vi "Set Helper Text.vi"(8 "error in (no error)":errorcluster, 10 "Helper Text":string, 11 "Filled Text Fields in":refnum<class "Filled Text Fields.lvclass">) -> (0 "error out":errorcluster, 3 "Filled Text Fields out":refnum<class "Filled Text Fields.lvclass">)   [LabVIEW 2017, in "Filled Text Fields.lvlib" / "Filled Text Fields.lvclass"]
uses:
  Filled Text Fields.lvclass
  Filled Text Fields.lvclass/Filled Text Fields.ctl
  Filled Text Fields Actor Messages/updateHelperText Msg/updateHelperText Msg.lvclass
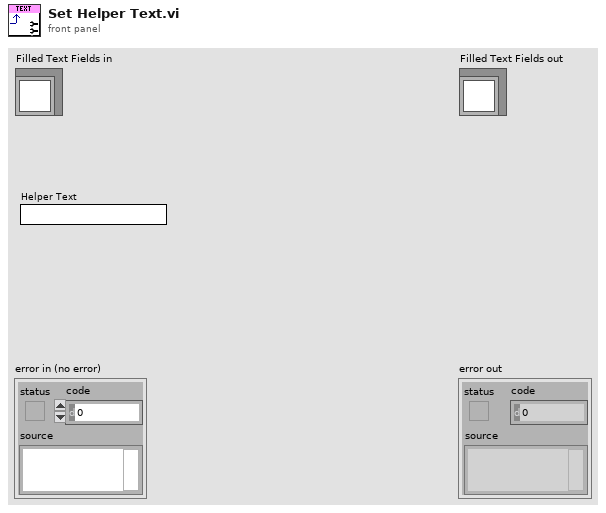
[diagram p1: front panel]
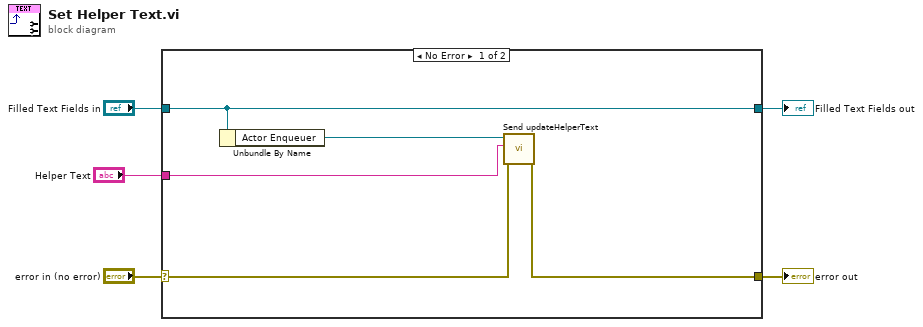
[diagram p0: block diagram]
diagram:
  n1 = case shown="No Error" "error in (no error)" {
    selector: "error in (no error)" -> [w7 w12]
    tunnel: [w8 w12] -> w4
    tunnel: [w10 w11] -> w2
    tunnel: "Filled Text Fields in" -> [w10 w11]
    tunnel: "Helper Text" -> [w6 _]
    frame No Error {
      n2 = Unbundle By Name(w10) -> ("Actor Enqueuer"=w9:refnum<class "Message Enqueuer.lvclass">)
      n3 = call "Send updateHelperText.vi"("error in (no error)"=w7, "Helper Text"=w6, "Message Enqueuer in"=w9) -> ("error out"=w8:errorcluster)  [unwired: 7 in, 1 out]
    }
    frame Error {
    }
  }
  "error out" <- w4
  "Filled Text Fields out" <- w2
